vi "Build_tdms_group_name.vi"(9 "SiPM Y":i32, 10 "SiPM X":i32, 11 "Date":string) -> (3 "Group_name":string)   [LabVIEW 2019]
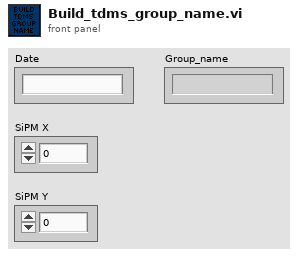
[diagram p1: front panel]
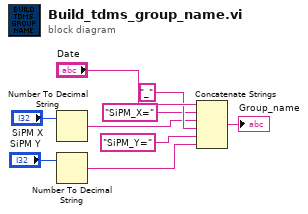
[diagram p0: block diagram]
diagram:
  n1 = Number To Decimal String(number="SiPM X") -> (decimal integer string=w4:string)  [unwired: 1 in]
  n2 = Number To Decimal String(number="SiPM Y") -> (decimal integer string=w7:string)  [unwired: 1 in]
  n3 = Concatenate Strings("Date", "SiPM_X=" ("group name in (Untitled)"), w4, "_" ("string"), "SiPM_Y=" ("group name in (Untitled)"), w7) -> (→"Group_name":string)
